vi "serial FPGA Main.vi"() -> ()   [LabVIEW 2009]
uses:
  <vilib>/rvi/DataTransferAndStorage/Container/XNode/niFpgaContainer.xnode
  <vilib>/rvi/FIFO/Fifo_Resource/nirvififoUniquifyingName.vi
panel:
  out "VectorNav Read: Char":u8
  out "VectorNav Read: New Data":bool
  in  "stop":bool
  in  "LIDAR Write: Char":u8
  in  "LIDAR Write: Data Written":bool
  out "LIDARRead: Char":u8
  out "LIDAR Read: New Data":bool
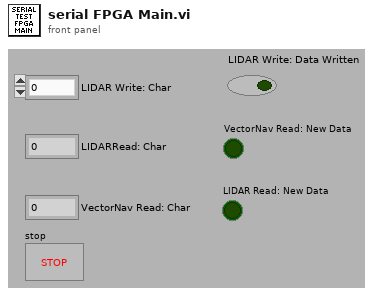
[diagram p1: front panel]
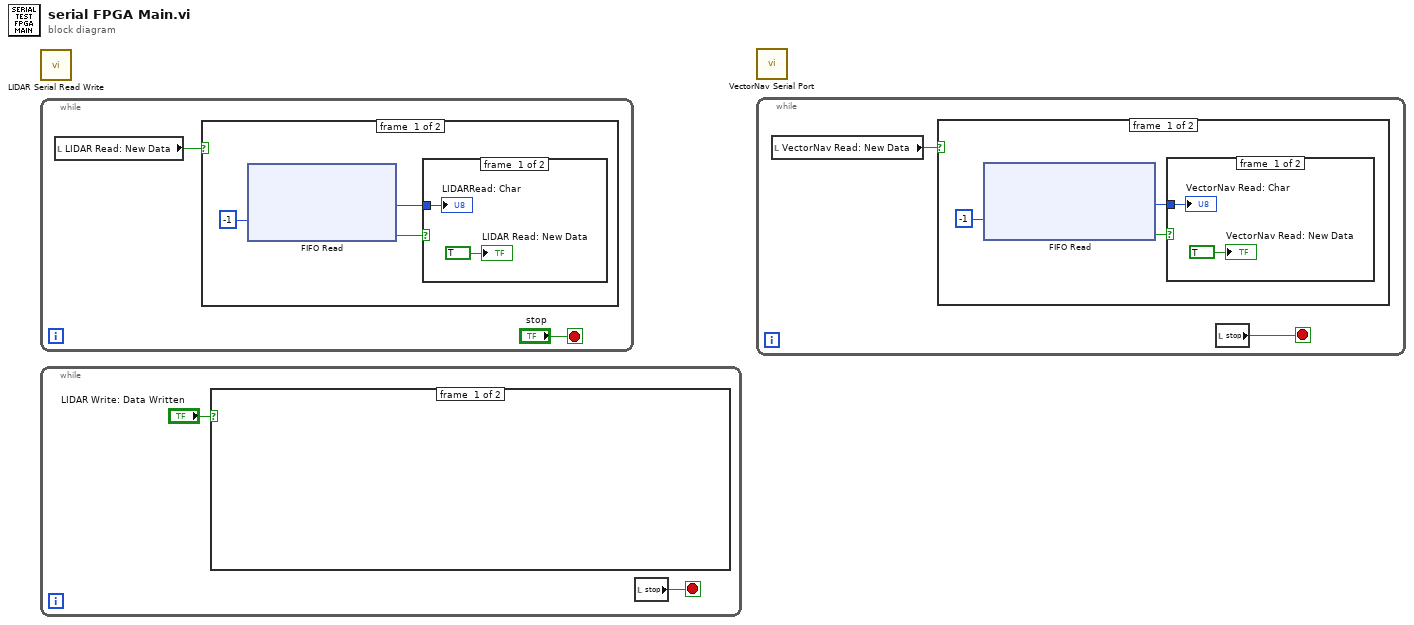
[diagram p0: block diagram]
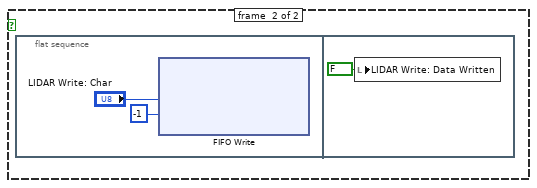
[diagram p6: hidden frame]
diagram:
  n1 = call "LIDAR Serial Read Write.vi"() -> ()  [unwired: 1 in]
  n2 = while {
    stop <- "stop" stop-if-true
    n3 = local read "LIDAR Read: New Data"() -> (w2:bool)
    n4 = case shown="False" w2 {
      frame #0 {
        n5 = xnode ("FIFO Read")("Timeout"=-1) -> ("Element"=w3:u8, "Timed Out?"=w4:bool)  [unwired: 1 in, 1 out]
        n6 = case shown="False" w4 {
          tunnel: w3 -> [w55 _]
          frame #0 {
            "LIDARRead: Char" <- w55
            "LIDAR Read: New Data" <- TRUE ("Read: New Data")
          }
          frame #1 {
          }
        }
      }
      frame #1 {
      }
    }
  }
  n7 = while {
    stop <- w56 stop-if-true
    n8 = case shown="True" "LIDAR Write: Data Written" {
      frame #0 {
      }
      frame #1 {
        n9 = flat-sequence {
          frame #0 {
            n10 = xnode ("FIFO Write")("Element"="LIDAR Write: Char", "Timeout"=-1) -> ()  [unwired: 1 in, 2 out]
          }
          frame #1 {
            n11 = local write "LIDAR Write: Data Written"(FALSE ("Write: Data Written")) -> ()
          }
        }
      }
    }
    n12 = local read "stop"() -> (w56:bool)
  }
  n13 = call "VectorNav Serial Port.vi"() -> ()  [unwired: 1 in]
  n14 = while {
    stop <- w109 stop-if-true
    n15 = local read "VectorNav Read: New Data"() -> (w110:bool)
    n16 = case shown="False" w110 {
      frame #0 {
        n17 = xnode ("FIFO Read")("Timeout"=-1) -> ("Element"=w111:u8, "Timed Out?"=w112:bool)  [unwired: 1 in, 1 out]
        n18 = case shown="False" w112 {
          tunnel: w111 -> [w163 _]
          frame #0 {
            "VectorNav Read: Char" <- w163
            "VectorNav Read: New Data" <- TRUE ("Read: New Data")
          }
          frame #1 {
          }
        }
      }
      frame #1 {
      }
    }
    n19 = local read "stop"() -> (w109:bool)
  }
